vi "1-Tap 10-Bit Camera with Frame Trigger (Host).vi"() -> ()   [LabVIEW 2012]
doc: "This is the host VI for the 1-Tap 10-Bit Camera with Frame Trigger example. This example demonstrates how to acquire images from a 1-tap, 10-bit, base configuration, Camera Link camera and display the images on the host. This example supports area scan and line scan cameras for both continuous and finite acquisitions.\n\nThis example also demonstrates the generation of a camera trigger using the Camera Control 1 signal on the Camera Link cable. The pulse width of this trigger can be customized to control the exposure of the camera, if supported. The source of the trigger can be software, via a button on the front panel, or a rising edge on the TTL In 0 signal.\n\nAdditionally, the example demonstrates the serial server, which allows third-party camera configuration utilities to communicate with the camera using the Camera Link serial interface while this VI is running."
uses:
  <vilib>/userdefined/High Color/nirio_resource_hc.ctl
  <vilib>/FPGAPlugInAG/PCIe-1473R/niLvFpga_Open_PCIe-1473R.vi
  <vilib>/rvi/interface/common/dynamic/niFpgaDynamicAddResources.vi
  <vilib>/FPGAPlugInAG/Dynamic/niLvFpga_Reset_Dynamic.vi
  <vilib>/Utility/error.llb/Error Cluster From Error Code.vi
  <vilib>/rvi/errors/niLvFpgaAdjustHostInterfaceError.vi
  <vilib>/FPGAPlugInAG/Dynamic/niLvFpga_Run_Dynamic.vi
  <vilib>/FPGAPlugInAG/Dynamic/niLvFpga_Close_Dynamic.vi
  <vilib>/rvi/interface/nirviOpenFPGA/nirviOpenFPGA.xnode
  FPGA Bitfiles/1-Tap10-BitCamer_FPGATarget_1-Tap10-BitCamer_1F5D4E78.lvbitx
  1-Tap 10-Bit Camera with Frame Trigger (FPGA).vi
  <vilib>/rvi/interface/nirviMethod/nirviMethod.xnode
  <vilib>/rvi/interface/nirviReadWriteControl/nirviReadWriteControl.xnode
  <vilib>/rvi/interface/nirviCloseFPGA/nirviCloseFPGA.xnode
  NiFpgaLv.dll
  <vilib>/rvi/interface/Simulation/niFpgaSimulationCallBeginRW.vi
  <vilib>/rvi/errors/niLvFpgaMergeErrorWithErrorCode.vi
  <vilib>/FPGAPlugInAG/Dynamic/niLvFpga_ConfigureFifo_Dynamic.vi
  <vilib>/FPGAPlugInAG/Dynamic/niLvFpga_StartFifo_Dynamic.vi
  <vilib>/FPGAPlugInAG/Dynamic/niLvFpga_ReadFifo_Dynamic.vi
panel:
  out "Acq In Progress":bool
  in  "Line Scan":bool
  in  "Frames To Acquire":u32=1 caption="Frames To Acquire\n(0 = infinite)"
  in  "Cancel":bool
  out "Acq'd Frame Width":u32
  in  "Stopped":bool
  in  "Trigger Pulse Width (us)":u32=1000
  in  "RIO Device":T1="RIO0"
  out "DMA Write Timeout":bool
  in  "Start Serial Server":bool=TRUE
  out "Frames Acq'd":u32
  out "Acq'd Frame Height":u32
  in  "Software Trigger":bool
  out "Image":T2(plugin-control)
  in  "Acquire":bool
  in  "Stop":bool
  in  "Image Height":u32=480 max=65535
  in  "Image Width":u32=640 max=65535
  out "Initialized":bool
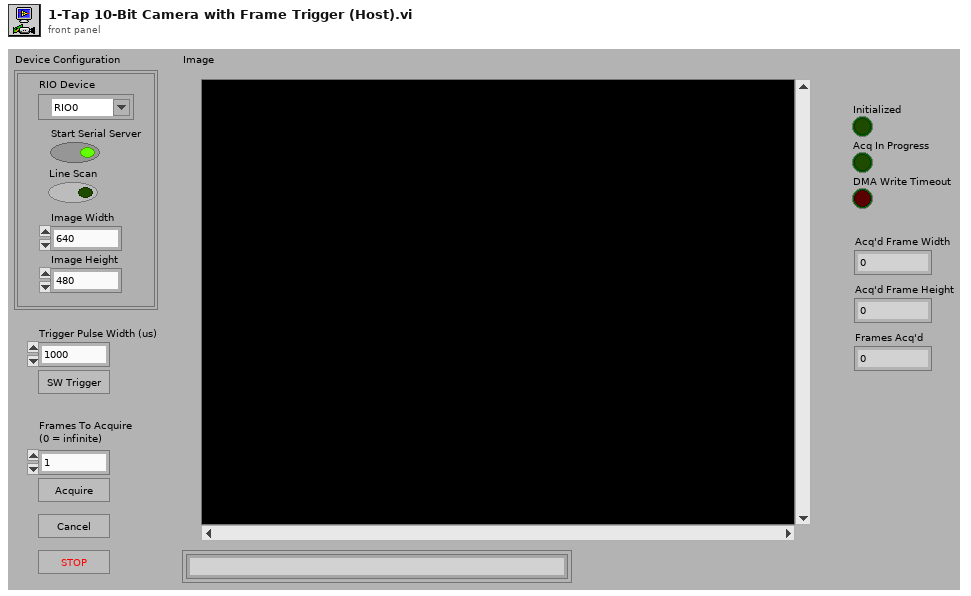
[diagram p1: front panel]
types:
  T1 = typedef "nirio_resource_hc.ctl" = tag
  T2 = typedef "IMAQ Image.ctl" = refnum<image>
  T3 = enum8{"Standard", "Basler 10-tap", "Vosskühler 10-tap"}
  T4 = typedef "Image Type" = u32
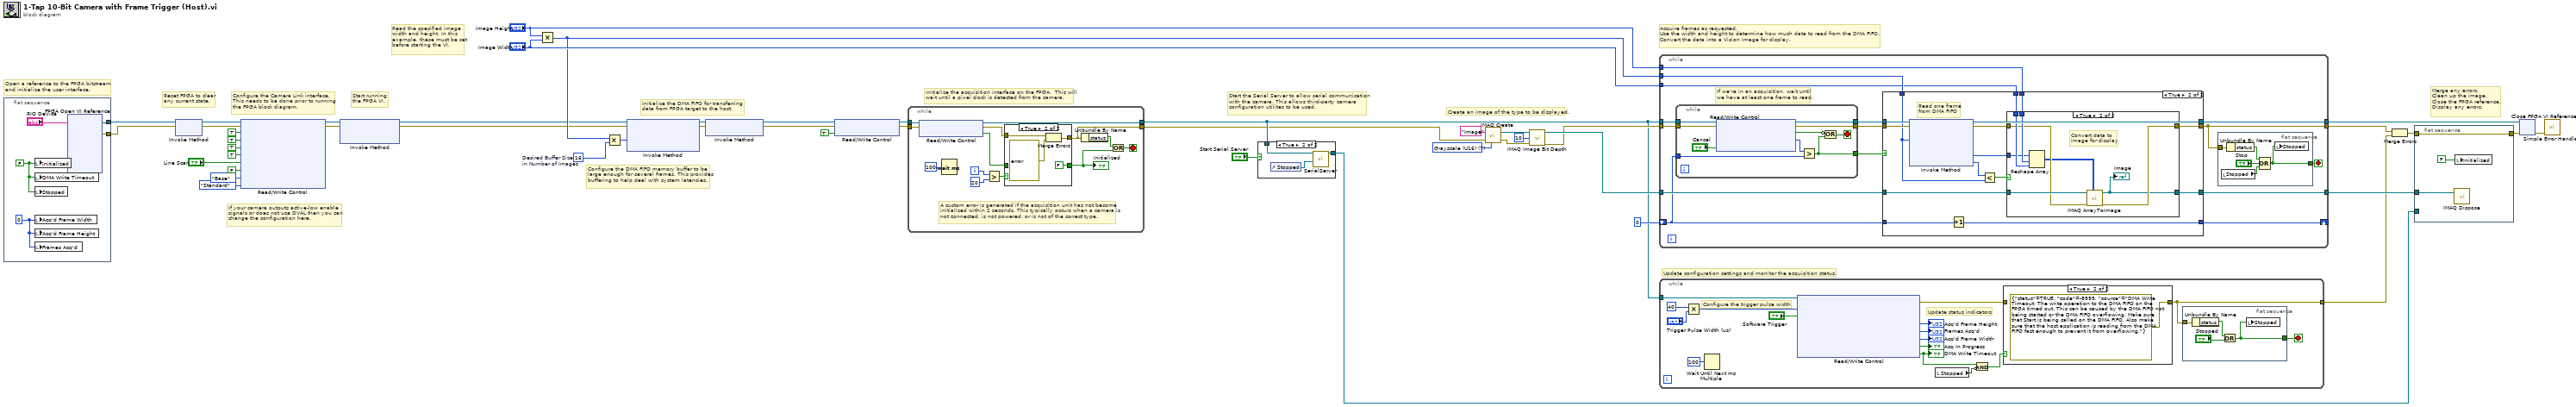
[diagram p0: block diagram]
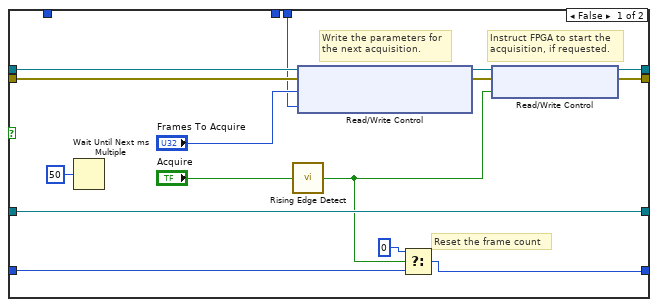
[diagram p4: hidden frame]
diagram:
  w43 = T4 7 items=["Grayscale (U8)", "Grayscale (I16)", "Grayscale (SGL)", "Complex (CSG)", "RGB (U32)", "HSL (U32)", "RGB (U64)", "Grayscale (U16)"] ("Image Type")
  w10 = u32 16  # Desired Buffer Size in Number of Images
  # "If your camera outputs active-low enable\nsignals or does not use DVAL then you can\nchange the configuration here."
  # "Configure the DMA FIFO memory buffer to be\nlarge enough for several frames. This provides\nbuffering to help deal with system latencies."
  # "Start running\nthe FPGA VI."
  # "Reset FPGA to clear\nany current state."
  # "Read the specified image\nwidth and height. In this\nexample, these must be set\nbefore starting the VI."
  # "Merge any errors.\nClean up the image.\nClose the FPGA reference.\nDisplay any errors."
  # "Acquire frames as requested.\nUse the width and height to determine how much data to read from the DMA FIFO.\nConvert the data into a Vision Image for display."
  # "Update configuration settings and monitor the acquisition status."
  # "Start the Serial Server to allow serial communication\nwith the camera. This allows third-party camera\nconfiguration utilites to be used."
  # "Create an image of the type to be displayed."
  # "Initialize the acquisition interface on the FPGA.  This will\nwait until a pixel clock is detected from the camera."
  # "Initialize the DMA FIFO for transferring\ndata from FPGA target to the host."
  # "Configure the Camera Link interface.\nThis needs to be done prior to running\nthe FPGA block diagram."
  # "Open a reference to the FPGA bitstream\nand initialize the user interface."
  n1 = flat-sequence {
    tunnel: [w49] -> w30
    tunnel: [w48] -> w47
    frame #0 {
      w52 = u32 0 ("Num Lines Acq'd")
      w51 = FALSE ("stop")
      n2 = local write "Initialized"(w51) -> ()
      n3 = local write "DMA Write Timeout"(w51) -> ()
      n4 = local write "Stopped"(w51) -> ()
      n5 = local write "Acq'd Frame Width"(w52) -> ()
      n6 = local write "Acq'd Frame Height"(w52) -> ()
      n7 = local write "Frames Acq'd"(w52) -> ()
      n8 = xnode "FPGA Open VI Reference"("resource name"="RIO Device") -> ("FPGA VI Reference Out"=w49:refnum<k20>, "error out"=w48:errorcluster)  [unwired: 1 in]
    }
  }
  n9 = xnode "Invoke Method"("FPGA VI Reference In"=w30, "error in"=w47) -> ("FPGA VI Reference Out"=w19:refnum<k20>, "error out"=w22:errorcluster)
  n10 = xnode "Read/Write Control"("FPGA VI Reference In"=w19, "error in"=w22, "CL Config.FVAL Active High"=TRUE ("IO Module Config.CL FVAL Active High"), "CL Config.LVAL Active High"=TRUE ("IO Module Config.CL LVAL Active High"), "CL Config.DVAL Active High"=TRUE ("IO Module Config.CL DVAL Active High"), "CL Config.Spare Active High"=TRUE ("IO Module Config.CL Spare Active High"), "CL Config.Line Scan"="Line Scan", "Acq Control.Ignore DVAL"=FALSE ("CL Config.Line Scan"), "CL Config.Configuration"=enum8{"Base", "Medium", "Full"}."Base", "CL Config.Signal Mapping"=T3."Standard") -> ("FPGA VI Reference Out"=w23:refnum<k20>, "error out"=w21:errorcluster)
  n11 = xnode "Invoke Method"("FPGA VI Reference In"=w23, "error in"=w21) -> ("FPGA VI Reference Out"=w2:refnum<k20>, "error out"=w1:errorcluster)  [unwired: 1 in]
  n12 = Multiply(x="Image Height", y="Image Width") -> (x*y=w5:u32)
  n13 = Multiply(x=w5, y=w10) -> (x*y=w13:u32)
  n14 = xnode "Invoke Method"("FPGA VI Reference In"=w2, "error in"=w1, "Requested Depth"=w13) -> ("FPGA VI Reference Out"=w29:refnum<k20>, "error out"=w28:errorcluster)  [unwired: 1 out]
  n15 = xnode "Invoke Method"("FPGA VI Reference In"=w29, "error in"=w28) -> ("FPGA VI Reference Out"=w14:refnum<k20>, "error out"=w27:errorcluster)
  n16 = xnode "Read/Write Control"("FPGA VI Reference In"=w14, "error in"=w27, "Acq Control.Initialize"=TRUE ("Arm Acquisition")) -> ("FPGA VI Reference Out"=w46:refnum<k20>, "error out"=w45:errorcluster)
  n17 = while {
    tunnel: w46 -> [w60]
    tunnel: w45 -> [w59]
    tunnel: [w58] -> w9
    tunnel: [w62] -> w8
    i -> [w54]
    stop <- w65 stop-if-true
    # "A custom error is generated if the acquisition unit has not become\ninitialized within 2 seconds. This typically occurs when a camera is\nnot connected, is not powered, or is not of the correct type."
    n18 = xnode "Read/Write Control"("FPGA VI Reference In"=w60, "error in"=w59) -> ("FPGA VI Reference Out"=w58:refnum<k20>, "error out"=w57:errorcluster, "Acq Status.Initialized"=w56:bool)
    n19 = Wait (ms)(milliseconds to wait=u32 100) -> ()  [unwired: 1 out]
    n20 = Greater?(x=w54, y=20) -> (0:w55:bool)
    n21 = case shown="True" w55 {
      tunnel: [w67 FALSE] -> w61
      tunnel: w56 -> [w67 _]
      tunnel: w57 -> [w66 w69]
      tunnel: [w66 w71] -> w62
      frame False {
      }
      frame True {
        n22 = Merge Errors(w69, errorcluster {"status"=TRUE, "code"=-8999, "source"="Acquisition Initialization: This error typically occurs when a camera is not properly connected, is not powered, or is not of the correct type."} ("error in")) -> (w71:errorcluster)
      }
    }
    "Initialized" <- w61
    n23 = Unbundle By Name(w62) -> ("status"=w64:bool)
    n24 = Or(x=w64, y=w61) -> (x .or. y?=w65:bool)
  }
  n25 = case shown="True" "Start Serial Server" {
    tunnel: [_ w72] -> w31
    tunnel: w9 -> [_ w73]
    frame False {
    }
    frame True {
      n26 = control-ref of="Stopped"() -> (w74:refnum<vi>)
      n27 = call "SerialServer.vi"("Stop Refnum"=w74, "FPGA VI Reference In"=w73) -> ("FPGA VI Reference Out"=w72:refnum<k20>)  [unwired: 5 in]
    }
  }
  n28 = call "IMAQ Create"("Image Name"="Image", "Image Type"=w43, "error in (no error)"=w8) -> ("New Image"=w39:T2, "error out"=w36:errorcluster)  [unwired: 2 in]
  n29 = call "IMAQ Image Bit Depth"("Image"=w39, "Bit Depth (0)"=u32 10, "error in (no error)"=w36) -> ("Image Out"=w37:T2, "error out"=w12:errorcluster)  [unwired: 10 in, 1 out]
  n30 = while {
    tunnel: w9 -> [w81]
    tunnel: w12 -> [w80]
    tunnel: w5 -> [w89]
    tunnel: "Image Height" -> [w88]
    tunnel: "Image Width" -> [w87]
    tunnel: w37 -> [w86]
    tunnel: [w84] -> w25
    tunnel: [w85] -> w42
    tunnel: [w82] -> w33
    shift-right: [w76] -> _
    shift-left: u32 0 -> [w75]
    stop <- w83 stop-if-true
    # "If we're in an acquisition, wait until \nwe have at least one frame to read."
    n31 = while {
      tunnel: w81 -> [w96]
      tunnel: w80 -> [w95]
      tunnel: [w93] -> w79
      tunnel: [w94] -> w78
      tunnel: w75 -> [w99]
      tunnel: [w97] -> w77
      stop <- w98 stop-if-true
      n32 = xnode "Read/Write Control"("FPGA VI Reference In"=w96, "error in"=w95, "Acq Control.Cancel Acq"="Cancel") -> ("FPGA VI Reference Out"=w94:refnum<k20>, "error out"=w93:errorcluster, "Acq Status.Acq In Progress"=w92:bool, "Acq Status.Frames Acq'd"=w91:u32)
      n33 = Greater?(x=w91, y=w99) -> (0:w97:bool)
      n34 = Compound Arithmetic op=OR(invert w92, w97) -> (w98:bool)
    }
    n35 = case shown="True" w77 {
      tunnel: w78 -> [w115 w127]
      tunnel: w79 -> [w114 w126]
      tunnel: w89 -> [_ w120]
      tunnel: w88 -> [w112 w134]
      tunnel: w87 -> [_ w133]
      tunnel: w86 -> [w119 w132]
      tunnel: [w108 w130] -> w84
      tunnel: [w111 w129] -> w85
      tunnel: [w119 w128] -> w82
      tunnel: w75 -> [w116 w125]
      tunnel: [w118 w124] -> w76
      frame False {
        # "Reset the frame count"
        # "Instruct FPGA to start the\nacquisition, if requested."
        # "Write the parameters for\nthe next acquisition."
        n36 = Wait Until Next ms Multiple(millisecond multiple=u32 50) -> ()  [unwired: 1 out]
        n37 = call "Rising Edge Detect.vi"("Input"="Acquire") -> ("Pulse"=w105:bool)  [unwired: 4 in]
        n38 = xnode "Read/Write Control"("FPGA VI Reference In"=w115, "error in"=w114, "Acq Control.Frames To Acq"="Frames To Acquire", "Acq Control.Line Scan Height"=w112) -> ("FPGA VI Reference Out"=w110:refnum<k20>, "error out"=w109:errorcluster)
        n39 = Select(t=u32 0, s=w105, f=w116) -> (s? t:f=w118:u32)
        n40 = xnode "Read/Write Control"("FPGA VI Reference In"=w110, "error in"=w109, "Acq Control.Acquire"=w105) -> ("FPGA VI Reference Out"=w111:refnum<k20>, "error out"=w108:errorcluster)
      }
      frame True {
        # "Read one frame\nfrom DMA FIFO"
        n41 = xnode "Invoke Method"("FPGA VI Reference In"=w127, "error in"=w126, "Number of Elements"=w120) -> ("FPGA VI Reference Out"=w129:refnum<k20>, "error out"=w131:errorcluster, "Data"=w123:u16[], "Elements Remaining"=w121:u32)  [unwired: 1 in]
        n42 = Increment(x=w125) -> (x+1=w124:u32)
        n43 = Less?(x=w121, y=w120) -> (x < y?=w122:bool)
        n44 = case shown="True" w122 {
          tunnel: w134 -> [_ w144]
          tunnel: w133 -> [_ w143]
          tunnel: w132 -> [w136 w142]
          tunnel: w131 -> [w135 w141]
          tunnel: [w135 w140] -> w130
          tunnel: [w136 w139] -> w128
          tunnel: w123 -> [_ w138]
          frame False {
            # "Do not display the image if we're\nfalling behind in the acquisition."
          }
          frame True {
            # "Convert data to\nimage for display"
            n45 = Reshape Array(w138, w144, w143) -> (w137:u16[][])
            n46 = call "IMAQ ArrayToImage"("Image Pixels (U16)"=w137, "error in (no error)"=w141, "Image"=w142) -> ("error out"=w140:errorcluster, "Image Out"=w139:T2)  [unwired: 7 in]
            "Image" <- w139
          }
        }
      }
    }
    n47 = flat-sequence {
      tunnel: w84 -> [w102]
      tunnel: [w101] -> w83
      frame #0 {
        n48 = local read "Stopped"() -> (w100:bool)
        n49 = Unbundle By Name(w102) -> ("status"=w103:bool)
        n50 = Compound Arithmetic op=OR(w103, "Stop", w100) -> (w101:bool)
        n51 = local write "Stopped"(w101) -> ()
      }
    }
  }
  n52 = while {
    tunnel: w9 -> [w157]
    tunnel: [w160] -> w24
    stop <- w159 stop-if-true
    # "Update status indicators"
    # "Configure the trigger pulse width"
    n53 = Multiply(x=u32 40, y="Trigger Pulse Width (us)") -> (x*y=w148:u32)
    n54 = Wait Until Next ms Multiple(millisecond multiple=u32 100) -> ()  [unwired: 1 out]
    n55 = xnode "Read/Write Control"("FPGA VI Reference In"=w157, "Trigger.Trigger Pulse Width (40 MHz Ticks)"=w148, "Trigger.Send Software Trigger"="Software Trigger") -> ("error out"=w156:errorcluster, "Acq Status.Lines Per Frame"=→"Acq'd Frame Height":u32, "Acq Status.Frames Acq'd"=→"Frames Acq'd":u32, "Acq Status.Clocks Per Line"=→"Acq'd Frame Width":u32, "Acq Status.Acq In Progress"=→"Acq In Progress":bool, "Acq Status.DMA Write Timeout"=w147:bool)  [unwired: 1 in, 1 out]
    "DMA Write Timeout" <- w147
    n56 = local read "Stopped"() -> (w146:bool)
    n57 = Compound Arithmetic op=AND(w147, invert w146) -> (w145:bool)
    n58 = case shown="True" w145 {
      tunnel: w156 -> [w165 _]
      tunnel: [w165 errorcluster {"status"=TRUE, "code"=-8999, "source"="DMA Write Timeout: The write operation to the DMA FIFO on the FPGA timed out. This can be caused by the DMA FIFO not being started or the DMA FIFO overflowing. Make sure that Start is being called on the DMA FIFO. Also make sure that the host application is reading from the DMA FIFO fast enough to prevent it from overflowing."} ("error out")] -> w160
      frame False {
      }
      frame True {
      }
    }
    n59 = flat-sequence {
      tunnel: w160 -> [w164]
      tunnel: [w162] -> w159
      frame #0 {
        n60 = Unbundle By Name(w164) -> ("status"=w163:bool)
        n61 = Or(x=w163, y="Stopped") -> (x .or. y?=w162:bool)
        n62 = local write "Stopped"(w162) -> ()
      }
    }
  }
  n63 = Merge Errors(w25, w24) -> (w26:errorcluster)
  n64 = flat-sequence {
    tunnel: w26 -> [w168]
    tunnel: [w168] -> w35
    tunnel: w33 -> [w169]
    tunnel: w31 -> [_]
    frame #0 {
      n65 = call "IMAQ Dispose"("Image"=w169) -> ()  [unwired: 5 in, 1 out]
      n66 = local write "Initialized"(FALSE ("Module Enabled")) -> ()
    }
  }
  n67 = xnode "Close FPGA VI Reference"("FPGA VI Reference In"=w42, "error in"=w35) -> ("error out"=w32:errorcluster)
  n68 = call <vilib>:"Simple Error Handler.vi"("error in (no error)"=w32) -> ()  [unwired: 4 in, 5 out]
